vi "PWM Input Read Frequency and DutyCycle.vi"(8 "error in (no error)":errorcluster, 11 "NI PWM Input in":refnum<class "NI PWM Input.lvclass">) -> (0 "error out":errorcluster, 1 "Duty Cycle":dbl[](array[numeric]), 2 "Frequency":dbl[](array[numeric]), 3 "NI PWM Input out":refnum<class "NI PWM Input.lvclass">)   [LabVIEW 2023, in "HardwareAbstractionLayer_LVOOP.lvlib" / "NI PWM Input.lvclass"]
uses:
  NI PWM Input.lvclass
  NI PWM Input.lvclass/NI PWM Input.ctl
  <vilib>/DAQmx/read.llb/DAQmx Read (Counter Pulse Freq 1 Chan 1 Samp).vi
  <vilib>/DAQmx/miscellaneous.llb/DAQmx Fill In Error Info.vi
  <vilib>/DAQmx/read.llb/DAQmx Read (Counter 1D Pulse Freq 1 Chan NSamp).vi
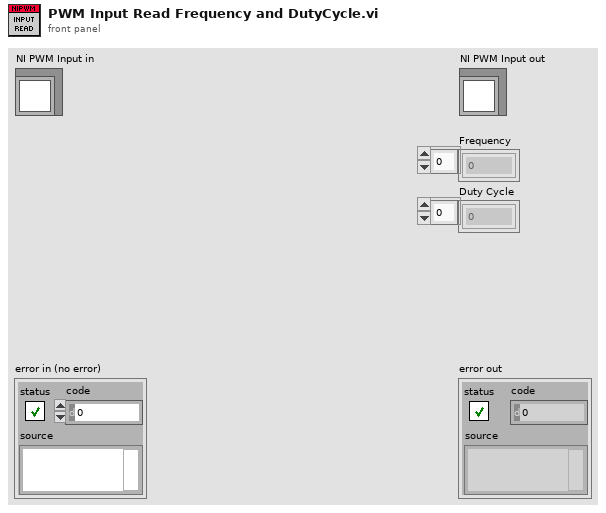
[diagram p1: front panel]
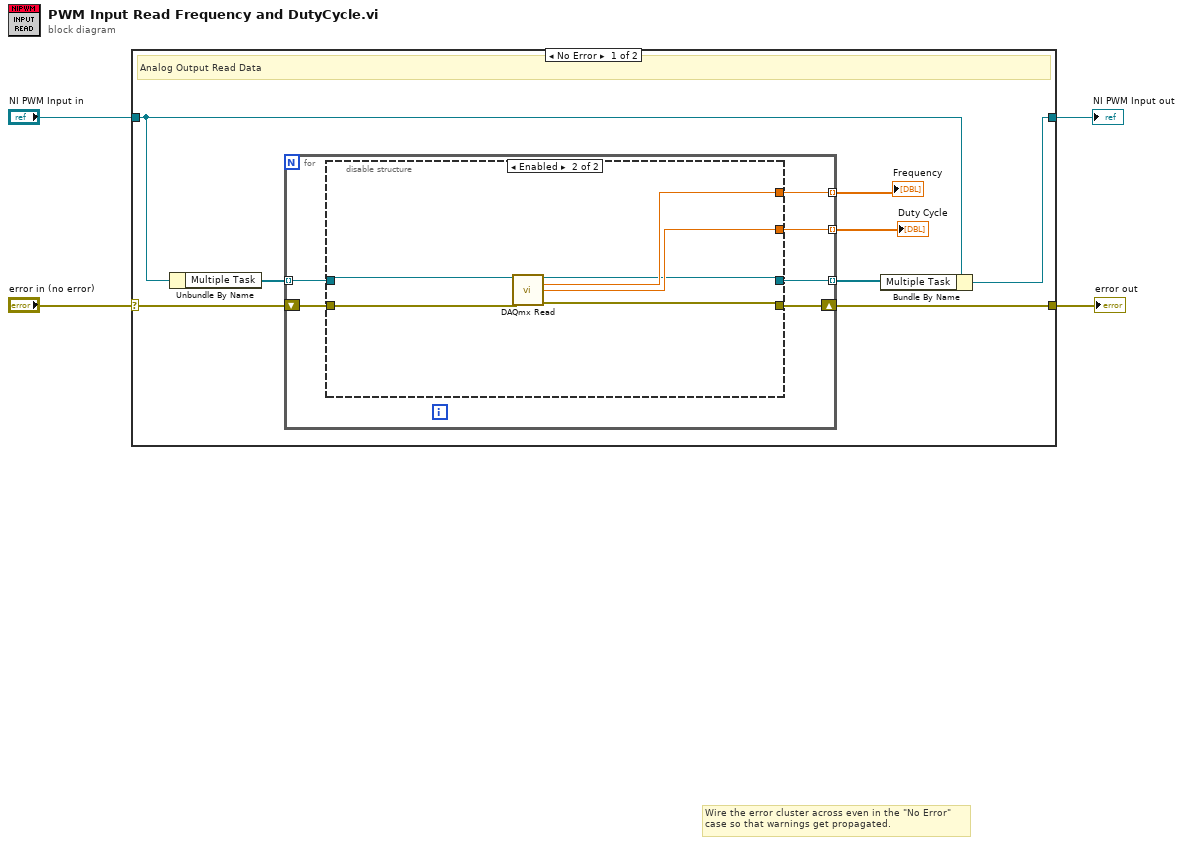
[diagram p0: block diagram]
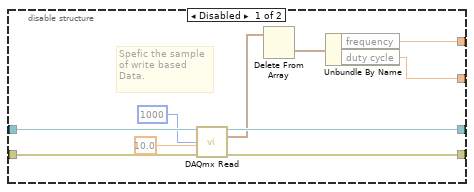
[diagram p2: hidden frame]
diagram:
  # "Wire the error cluster across even in the \"No Error\"\ncase so that warnings get propagated."
  n1 = case shown="No Error" "error in (no error)" {
    selector: "error in (no error)" -> [w12 w36]
    tunnel: [w11 w36] -> w3
    tunnel: [w9 w35] -> w1
    tunnel: "NI PWM Input in" -> [w10 w35]
    frame No Error {
      # "Analog Output Read Data"
      n2 = Unbundle By Name(w10) -> ("Multiple Task"=w8:refnum<k21>[])
      n3 = for {
        shift-right: [w17] -> w11
        shift-left: w12 -> [w18]
        tunnel: w8 -> [w16] mode=indexing
        tunnel: [w15] -> w7 mode=indexing
        tunnel: [w14] -> w6 mode=indexing
        tunnel: [w13] -> w5 mode=indexing
        n4 = disable-structure shown="Enabled" {
          disable-tunnel: w18 -> [w28 w33]
          disable-tunnel: [w27 w29] -> w17
          disable-tunnel: w16 -> [w26 w34]
          disable-tunnel: [w25 w30] -> w15
          disable-tunnel: [w21 w32] -> w14
          disable-tunnel: [w20 w31] -> w13
          frame Disabled {
            # "Spefic the sample of write based Data."
            n5 = call-poly <vilib>:"DAQmx Read.vi"("task/channels in"=w26, "number of samples per channel"=1000, "timeout"=10.0, "error in"=w28) -> ("task out"=w25:refnum<k21>, "data"=w23:cluster{"duty cycle":dbl, "frequency":dbl}[], "error out"=w27:errorcluster)  [unwired: 9 in]
            n6 = Delete From Array(array=w23) -> (deleted portion=w22:cluster{"duty cycle":dbl, "frequency":dbl})  [unwired: 2 in, 1 out]
            n7 = Unbundle By Name(w22) -> ("frequency"=w21:dbl, "duty cycle"=w20:dbl)
          }
          frame Enabled {
            n8 = call-poly <vilib>:"DAQmx Read.vi"("task/channels in"=w34, "error in"=w33) -> ("task out"=w30:refnum<k21>, "frequency"=w32:dbl, "duty cycle"=w31:dbl, "error out"=w29:errorcluster)  [unwired: 10 in]
          }
        }
      }
      "Frequency" <- w6
      "Duty Cycle" <- w5
      n9 = Bundle By Name(cluster=w10, "Multiple Task"=w7) -> (w9:refnum<class "NI PWM Input.lvclass">)
    }
    frame Error {
    }
  }
  "error out" <- w3
  "NI PWM Input out" <- w1
